vi "Image Coordinet.vi"(8 "error in (no error)":errorcluster, 9 "Out":T1(array[cluster]), 10 "index of element":i32, 11 "Picture in":refnum<vi>) -> (0 "error out":errorcluster)   [LabVIEW 2015]
uses:
  <vilib>/Utility/miscctls.llb/LVPointTypeDef.ctl
  <vilib>/Utility/miscctls.llb/LVBoundsTypeDef.ctl
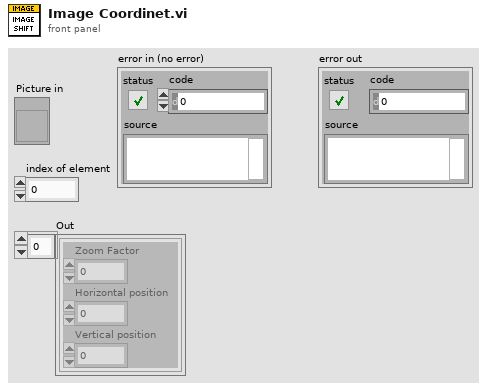
[diagram p1: front panel]
types:
  T1 = cluster{"Zoom Factor":sgl, "Horizontal position":sgl, "Vertical position":sgl}[]
  T2 = typedef "LVBoundsTypeDef.ctl" = cluster{"Width":u32, "Height":u32}
  T3 = typedef "LVPointTypeDef.ctl" = cluster{"Horizontal":i16, "Vertical":i16}
  T4 = cluster{"Zoom Factor":sgl, "Horizontal position":sgl, "Vertical position":sgl}
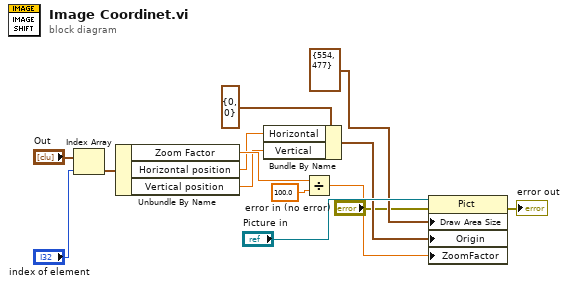
[diagram p0: block diagram]
diagram:
  n1 = Index Array(array="Out", index="index of element") -> (element=w6:T4)
  n2 = Unbundle By Name(w6) -> ("Zoom Factor"=w10:sgl, "Horizontal position"=w4:sgl, "Vertical position"=w3:sgl)
  n3 = Bundle By Name(cluster=T3 {"Horizontal"=0, "Vertical"=0} ("Origin"), "Horizontal"=w4, "Vertical"=w3) -> (w12:T3)
  n4 = Divide(x=w10, y=sgl 100.0 ("x")) -> (x/y=w13:sgl)
  n5 = property class="Pict"(reference="Picture in", error in="error in (no error)", "Draw Area Size"=T2 {"Width"=554, "Height"=477}, "Origin"=w12, "ZoomFactor"=w13) -> (error out=→"error out":errorcluster)  [unwired: 1 out]
